vi "Main.vi"() -> ()   [LabVIEW 2014]
uses:
  SubVIs/Type Defs/State.ctl
  SubVIs/Type Defs/Note Definition.ctl
  SubVIs/Type Defs/Clef.ctl
panel:
  in  "Landmark C's":bool
  out "value":u8
  out "Score":i32=23 format="%3.0f"
  out "2D Picture":picture
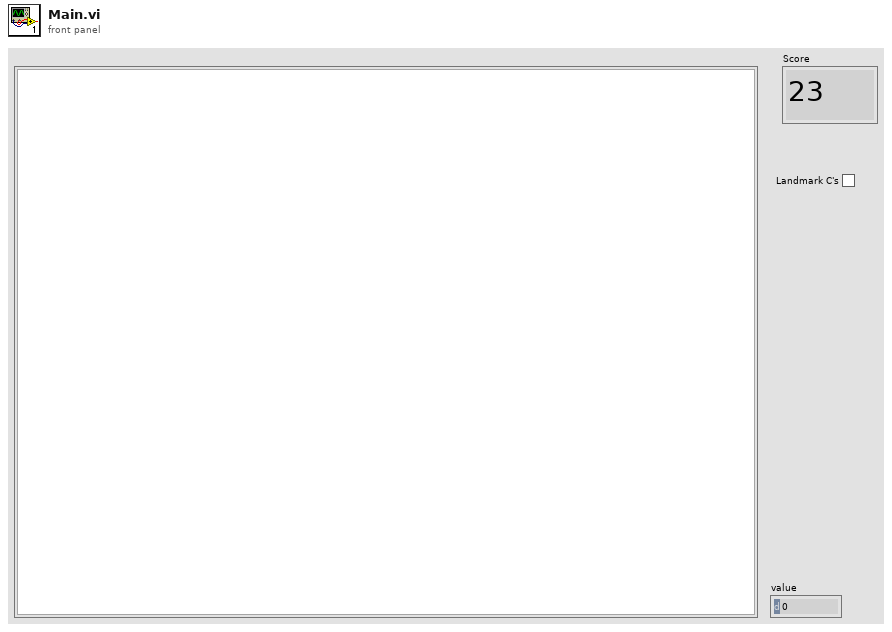
[diagram p1: front panel]
types:
  T1 = typedef "Note Definition.ctl" = cluster{"Clef":T2, "Note Number":i16}
  T2 = typedef "Clef.ctl" = enum16{"Treble", "Bass"}
  T3 = typedef "State.ctl" = enum16{"Initialize", "Load Set", "Idle", "Select Random Note"}
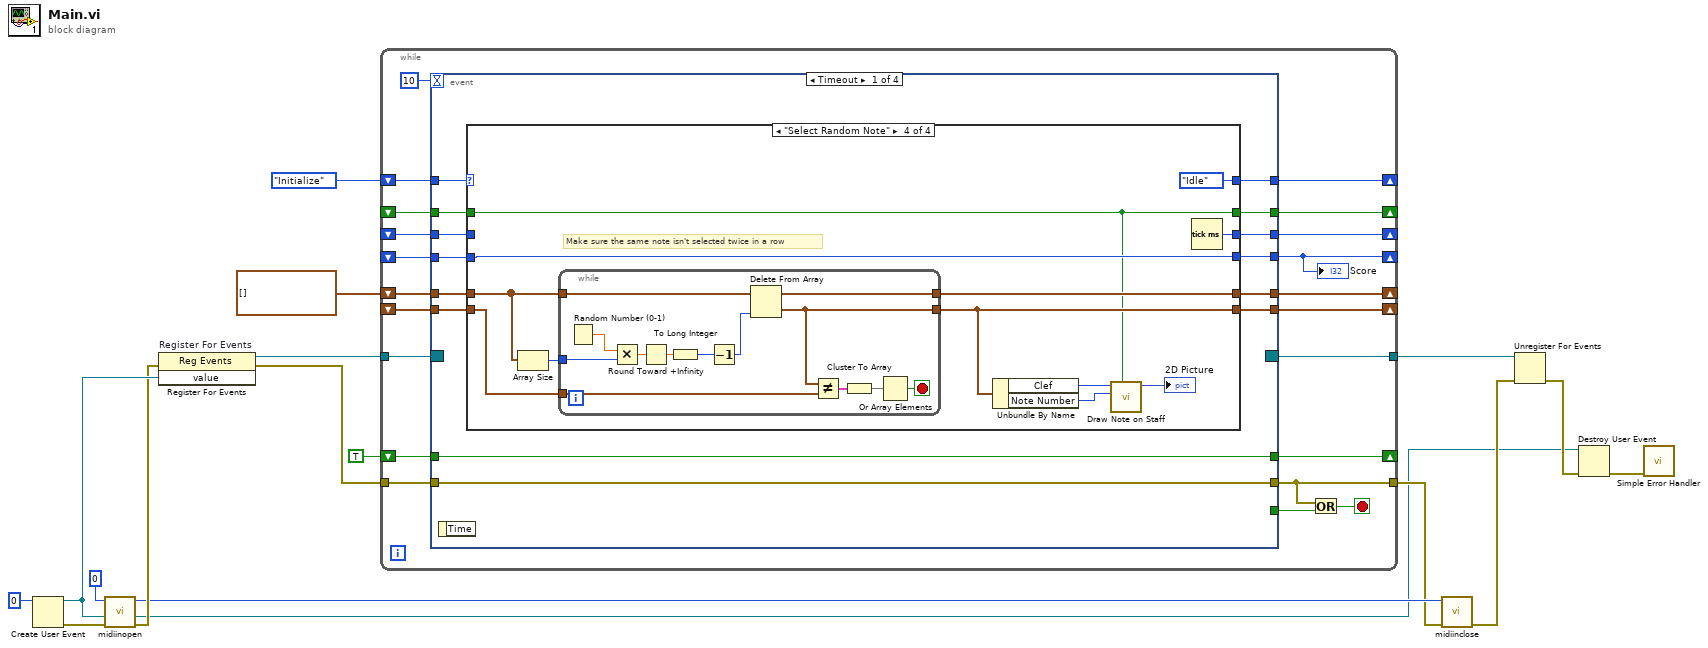
[diagram p0: block diagram]
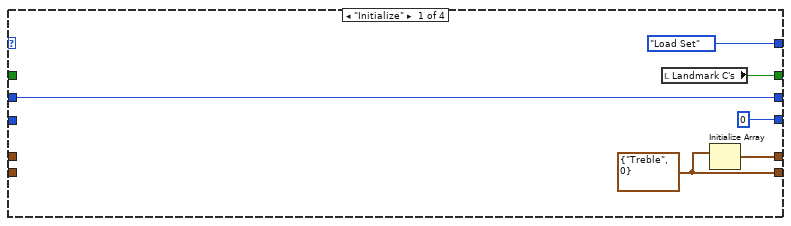
[diagram p2: hidden frame]
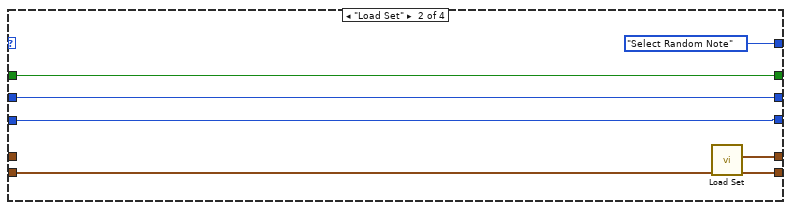
[diagram p3: hidden frame]
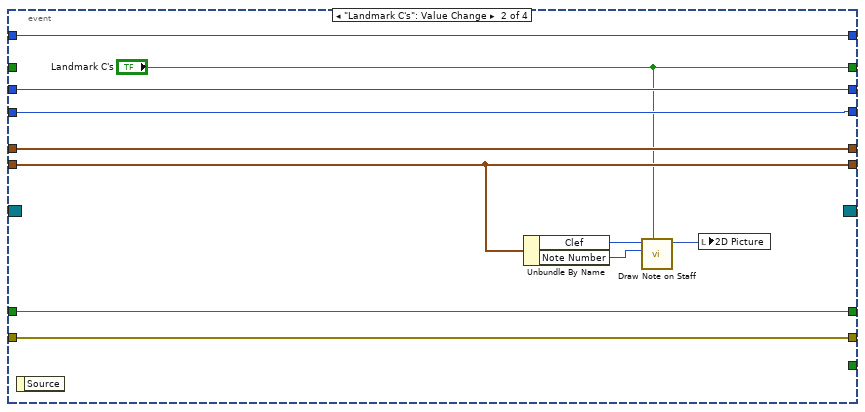
[diagram p5: hidden frame]
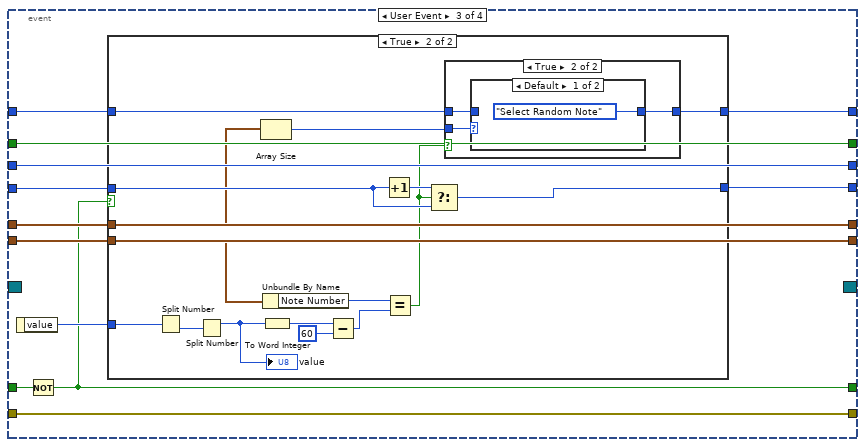
[diagram p6: hidden frame]
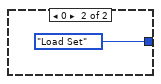
[diagram p9: hidden frame]
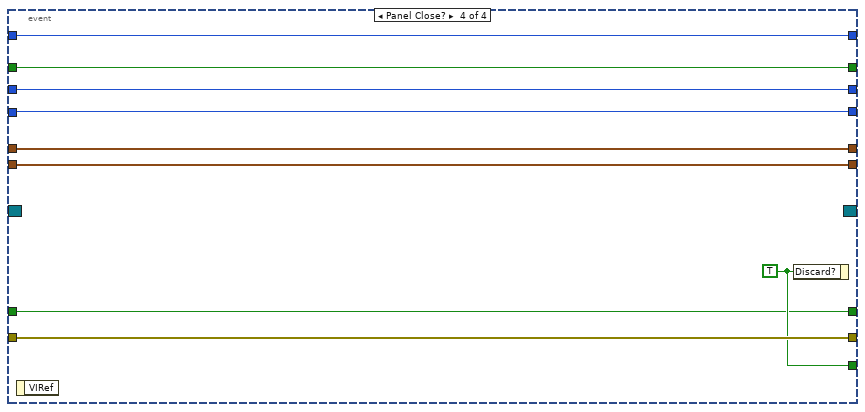
[diagram p10: hidden frame]
diagram:
  n1 = Create User Event(user event datatype=0 ("value")) -> (user event=w15:refnum<user-event>, error out=w10:errorcluster)  [unwired: 1 in]
  n2 = call "midiinopen.vi"("error in (no error)"=w10, "value"=w15, "MIDI Input Device"=0) -> ("error out"=w9:errorcluster, "value out"=w3:refnum<user-event>, "hmidiin"=w8:i32)  [unwired: 1 in, 1 out]
  n3 = register-events "Register For Events"(error in=w9, w15) -> (reference out=w12:refnum<event-registration>, error out=w7:errorcluster)  [unwired: 1 in]
  n4 = while {
    shift-right: [w37] -> _
    shift-left: T1[] [] ("Set") -> [w36]
    shift-right: [w35] -> _
    shift-left: State."Initialize" -> [w34]
    shift-right: [w33] -> _
    shift-left: _ -> [w32]
    shift-right: [w31] -> _
    shift-left: _ -> [w30]
    shift-right: [w18] -> _
    shift-left: _ -> [w29]
    tunnel: w12 -> [w28]
    tunnel: w7 -> [w27]
    tunnel: [w24] -> w6
    tunnel: [w26] -> w5
    shift-right: [w21] -> _
    shift-left: TRUE -> [w22]
    shift-right: [w20] -> _
    shift-left: _ -> [w19]
    stop <- w25 stop-if-true
    n5 = event shown="[0] Timeout" {
      selector: w28 -> [_ _ _ _]
      dyn-events: [_ _ _ _] -> w26
      timeout: 10 -> [_ _ _ _]
      tunnel: w34 -> [w52 w105 w116 w150]
      tunnel: [w51 w103 w110 w147] -> w37
      tunnel: w36 -> [w50 w103 w110 w147]
      tunnel: [w49 w105 w115 w150] -> w35
      tunnel: [w48 w97 w109 w146] -> w33
      tunnel: w32 -> [w47 w97 w109 w146]
      tunnel: [w46 w106 w111 w149] -> w31
      tunnel: w30 -> [w45 w106 w111 w149]
      tunnel: [w44 w104 w117 w148] -> w18
      tunnel: w29 -> [w43 w104 w118 w148]
      tunnel: w27 -> [w42 w101 w113 w151]
      tunnel: [w42 w101 w113 w151] -> w24
      tunnel: [_ _ _ w145] -> w23
      tunnel: w22 -> [w41 w102 w112 w144]
      tunnel: [w41 w102 w108 w144] -> w21
      tunnel: [w39 "Landmark C's" w107 w143] -> w20
      tunnel: w19 -> [w40 _ w107 w143]
      event Timeout {
        n6 = event-data() -> ()  [unwired: 1 in, 1 out]
        n7 = case shown="\"Select Random Note\"" w52 {
          selector: w52 -> [_ _ w70 _]
          tunnel: [w54 w61 w69 w82] -> w51
          tunnel: w50 -> [_ _ w69 w74]
          tunnel: [State."Load Set" State."Select Random Note" w70 State."Idle"] -> w49
          tunnel: [w55 w60 w66 w77] -> w48
          tunnel: w47 -> [_ w60 w66 w72]
          tunnel: [w56 w63 w68 w76] -> w46
          tunnel: w45 -> [w56 w63 w68 _]
          tunnel: [0 w62 w67 w75] -> w44
          tunnel: w43 -> [_ w62 w67 w75]
          tunnel: w40 -> [_ w59 w65 w71]
          tunnel: [w53 w59 w65 w71] -> w39
          frame "Initialize" {
            w55 = T1 {"Clef"=enum."Treble", "Note Number"=0} ("Note Def 2")
            n8 = local read "Landmark C's"() -> (w53:bool)
            n9 = Initialize Array(w55) -> (w54:T1[])  [unwired: 1 in]
          }
          frame "Load Set" {
            n10 = call "Load Set.vi"() -> ("Set"=w61:T1[])  [unwired: 11 in]
          }
          frame "Idle" {
          }
          frame "Select Random Note" {
            # "Make sure the same note isn't selected twice in a row"
            n11 = Array Size(array=w74) -> (size(s)=w73:i32)
            n12 = while {
              tunnel: [w87] -> w77
              tunnel: w73 -> [w88]
              tunnel: w72 -> [w86]
              tunnel: w74 -> [w89]
              tunnel: [w90] -> w82
              stop <- w83 stop-if-true
              n13 = Random Number (0-1)() -> (number: 0 to 1=w92:dbl)
              n14 = Multiply(x=w92, y=w88) -> (x*y=w93:dbl)
              n15 = Round Toward +Infinity(x=w93) -> (ceil(x): smallest int >= x=w94:dbl)
              n16 = To Long Integer(number=w94) -> (32bit integer=w95:i32)
              n17 = Decrement(x=w95) -> (x-1=w91:i32)
              n18 = Delete From Array(array=w89, index=w91) -> (deleted portion=w87:T1, array with subset deleted=w90:T1[])  [unwired: 1 in]
              n19 = Not Equal?(x=w87, y=w86) -> (x != y?=w85:cluster{"Clef":bool, "Note Number":bool})
              n20 = Cluster To Array(cluster=w85) -> (array=w84:bool[])
              n21 = Or Array Elements(Boolean array=w84) -> (logical OR=w83:bool)
            }
            n22 = Unbundle By Name(w77) -> ("Clef"=w80:T2, "Note Number"=w81:i16)
            n23 = call "Draw Note on Staff.vi"("Landmark C's"=w71, "Note Number"=w81, "Clef"=w80) -> ("picture out"=→"2D Picture":picture)  [unwired: 8 in]
            n24 = Tick Count (ms)() -> (millisecond timer value=w76:u32)
          }
        }
      }
      event "Landmark C's": Value Change {
        n25 = event-data() -> ()  [unwired: 1 in, 1 out]
        n26 = Unbundle By Name(w97) -> ("Clef"=w99:T2, "Note Number"=w100:i16)
        n27 = call "Draw Note on Staff.vi"("Landmark C's"="Landmark C's", "Note Number"=w100, "Clef"=w99) -> ("picture out"=w98:picture)  [unwired: 8 in]
        n28 = local write "2D Picture"(w98) -> ()
      }
      event User Event {
        n29 = event-data() -> ("value"=w114:i32)  [unwired: 1 in]
        n30 = Not(x=w112) -> (.not. x?=w108:bool)
        n31 = case shown="True" w108 {
          tunnel: w118 -> [w120 w136]
          tunnel: [w120 w135] -> w117
          tunnel: w116 -> [w119 w134]
          tunnel: [w119 w133] -> w115
          tunnel: w114 -> [_ w132]
          tunnel: w110 -> [_ w131]
          tunnel: w109 -> [_ w130]
          frame False {
          }
          frame True {
            n32 = Split Number(x=w132) -> (lo(x)=w122:u16)  [unwired: 1 out]
            n33 = Split Number(x=w122) -> (hi(x)=w121:u8)  [unwired: 1 out]
            "value" <- w121
            n34 = Array Size(array=w131) -> (size(s)=w127:i32)
            n35 = To Word Integer(number=w121) -> (16bit integer=w125:i16)
            n36 = Unbundle By Name(w130) -> ("Note Number"=w123:i16)
            n37 = Subtract(x=w125, y=i16 60) -> (x-y=w126:i16)
            n38 = Increment(x=w136) -> (x+1=w129:i32)
            n39 = Equal?(x=w123, y=w126) -> (x = y?=w128:bool)
            n40 = Select(t=w129, s=w128, f=w136) -> (s? t:f=w135:i32)
            n41 = case shown="True" w128 {
              tunnel: w134 -> [w137 w140]
              tunnel: w127 -> [_ w139]
              tunnel: [w137 w138] -> w133
              frame False {
              }
              frame True {
                n42 = case shown="Default" w139 {
                  tunnel: w140 -> [_ _]
                  tunnel: [State."Select Random Note" ("t") State."Load Set" ("t")] -> w138
                  frame Default {
                  }
                  frame 0 {
                  }
                }
              }
            }
          }
        }
      }
      event Panel Close? {
        w145 = TRUE ("Discard?")
        n43 = event-data() -> ()  [unwired: 1 in, 1 out]
        n44 = event-data("Discard?"=w145) -> ()  [unwired: 1 in, 1 out]
      }
    }
    "Score" <- w18
    n45 = Or(x=w24, y=w23) -> (x .or. y?=w25:bool)
  }
  n46 = call "midiinclose.vi"("error in (no error)"=w6, "hmidiin"=w8) -> ("error out"=w4:errorcluster)  [unwired: 4 in, 1 out]
  n47 = Unregister For Events ("Unregister\nFor Events")(event registration refnum=w5, error in=w4) -> (error out=w11:errorcluster)
  n48 = Destroy User Event ("Destroy\nUser Event")(user event=w3, error in=w11) -> (error out=w2:errorcluster)
  n49 = call <vilib>:"Simple Error Handler.vi"("error in (no error)"=w2) -> ()  [unwired: 4 in, 5 out]
